vi "example.vi"() -> ()   [LabVIEW 2014]
uses:
  <vilib>/NI/TBM Modules/Sequencer/module/execution/Simple Sequencer TBM runtime.lvclass
  Code/3D Gears Demo/Source Code/actions/dwell/Dwell Config.lvclass
  <vilib>/NI/TBM Modules/Sequencer/module/configuration/Simple Sequencer TBM configuration.lvclass
  <vilib>/NI/TBM Modules/Sequencer/module/configuration/sequence definition.ctl
  <vilib>/NI/TBM Modules/Sequencer/sequencer parent classes/sequencer config parent/base TBM sequencer configuration.lvclass
  <vilib>/NI/Tag Bus Module Framework/channel/TBM channel.lvclass
  <vilib>/NI/Tag Bus/tag/Data Type.ctl
  <vilib>/NI/Tag Bus/tag/tag descriptor.lvclass
  <vilib>/NI/Tag Bus Module Framework/channel/channel classification.ctl
  <vilib>/NI/TBM Modules/Sequencer/sequencer parent classes/action configuration parent/action configuration.lvclass
  Code/3D Gears Demo/Source Code/actions/toggle/configuration/Toggle Config.lvclass
  Code/3D Gears Demo/Source Code/actions/dwell/runtime/Dwell.lvclass
  Code/3D Gears Demo/Source Code/actions/toggle/runtime/Toggle.lvclass
panel:
  out "error out":errorcluster
  in  "stop":bool
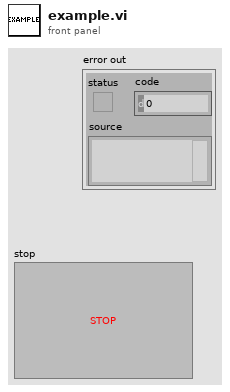
[diagram p1: front panel]
types:
  T1 = typedef "TBM channel.lvclass/channel classification.ctl" = enum16{"input data", "output data", "processing parameter", "processing result"}
  T2 = typedef "tag bus.lvlib/tag descriptor.lvclass/Data Type.ctl" = enum16{"Double", "Single", "I64", "I32", "I16", "I8", "U64", "U32", "U16", "U8", "Boolean", "String", "Array of Double", "Array of Single", "Array of I64", "Array of I32", "Array of I16", "Array of I8", "Array of U64", "Array of U32", "Array of U16", "Array of U8", "Array of Boolean", "Array of String"}
  T3 = typedef "Simple Sequencer TBM configuration.lvclass/sequence definition.ctl" = cluster{"sequence name":string, "action configs":refnum<class "action configuration.lvclass">[]}
  T4 = typedef "TBM channel.lvclass/data tables.ctl" = cluster{"input data":T5, "processing parameter":T5, "processing result":T5, "output data":T5}
  T5 = typedef "tag bus.lvlib/dictionary table pair.ctl" = cluster{"data dictionary":refnum<class "data dictionary.lvclass">, "data table":T6}
  T6 = typedef "tag bus.lvlib/data table.lvlib/data table.ctl" = cluster{"Double":dbl[], "Single":sgl[], "I64":i64[], "I32":i32[], "I16":i16[], "I8":i8[], "U64":u64[], "U32":u32[], "U16":u16[], "U8":u8[], "Boolean":bool[], "String":string[], "Array of Double":cluster{"DBL Array":dbl[]}[], "Array of Single":cluster{"SGL Array":sgl[]}[], "Array of I64":cluster{"I64 Array":i64[]}[], "Array of I32":cluster{"I32 Array":i32[]}[], "Array of I16":cluster{"I16 Array":i16[]}[], "Array of I8":cluster{"I8 Array":i8[]}[], "Array of U64":cluster{"U64 Array":u64[]}[], "Array of U32":cluster{"U32 Array":u32[]}[], "Array of U16":cluster{"U16 Array":u16[]}[], "Array of U8":cluster{"U8 Array":u8[]}[], "Array of Boolean":cluster{"Boolean Array":bool[]}[], "Array of String":cluster{"String Array":string[]}[]}
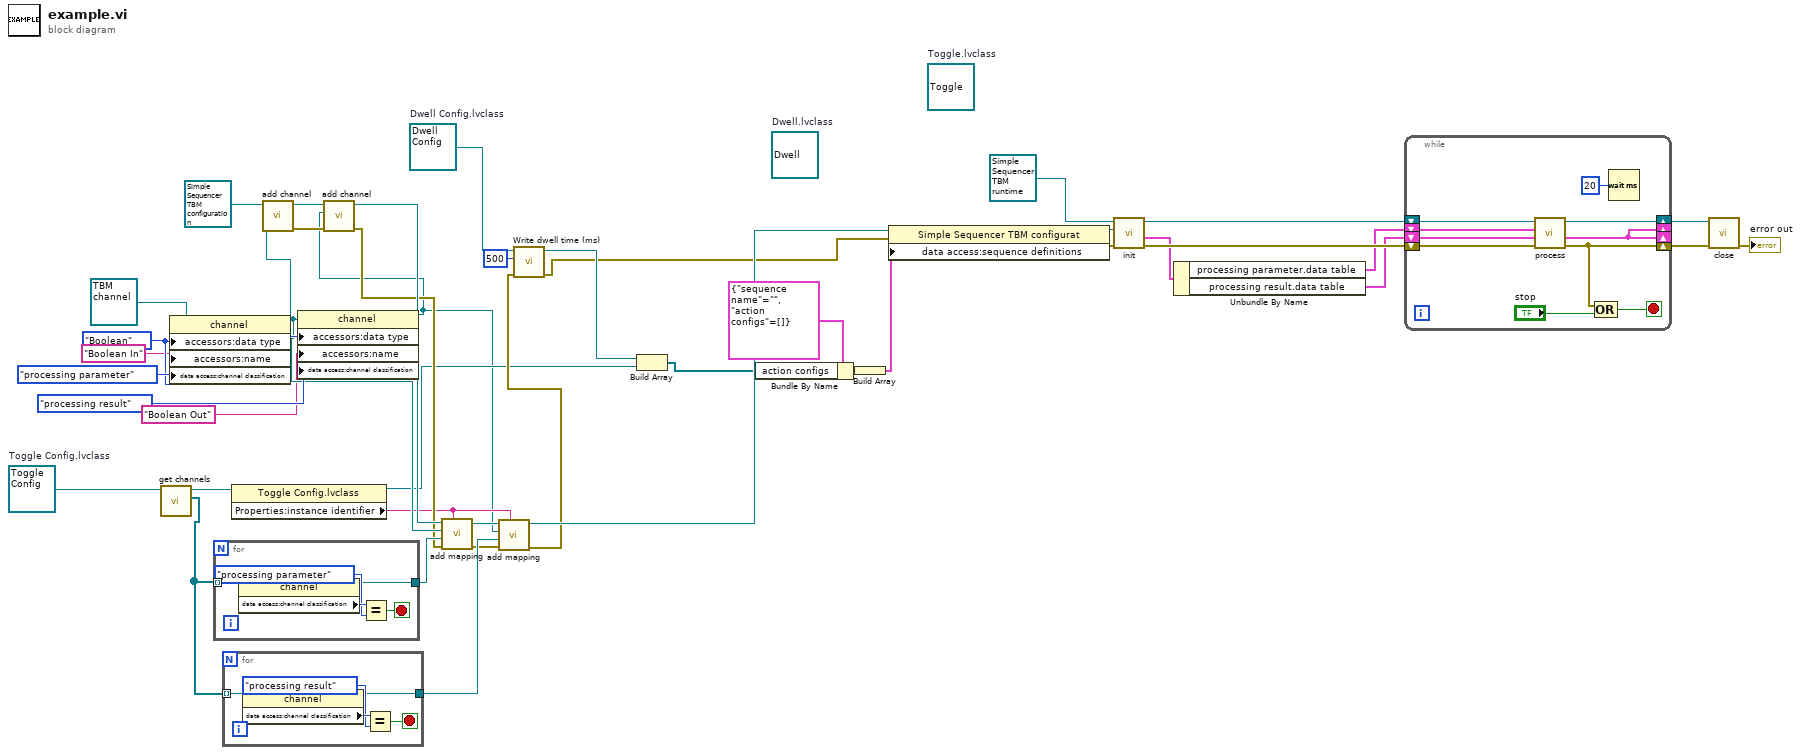
[diagram p0: block diagram]
diagram:
  (unwired) refnum<class "Toggle.lvclass"> refnum  # Toggle.lvclass
  (unwired) refnum<class "Dwell.lvclass"> refnum  # Dwell.lvclass
  w1 = refnum<class "Dwell Config.lvclass"> refnum  # Dwell Config.lvclass
  w2 = refnum<class "Toggle Config.lvclass"> refnum  # Toggle Config.lvclass
  w24 = Data_Type."Boolean" ("data type")
  n1 = call-dynamic "get channels.vi"("ActionCfg_Toggle in"=w2) -> ("action channels"=w13:refnum<class "TBM channel.lvclass">[], "ActionCfg_Toggle out"=w19:refnum<class "Toggle Config.lvclass">)  [unwired: 8 in, 1 out]
  n2 = property class="channel"(reference=refnum<class "TBM channel.lvclass"> refnum ("channel descriptor"), "accessors:data type"=w24, "accessors:name"="Boolean In" ("name"), "data access:channel classification"=channel_classification."processing parameter" ("channel classification")) -> (reference out=w18:refnum<class "TBM channel.lvclass">)  [unwired: 1 in, 1 out]
  n3 = for {
    tunnel: w13 -> [w48] mode=indexing
    tunnel: [w44] -> w17
    stop <- w45 stop-if-true
    n4 = property class="channel"(reference=w48) -> (reference out=w44:refnum<class "TBM channel.lvclass">, "data access:channel classification"=w47:T1)  [unwired: 1 in, 1 out]
    n5 = Equal?(x=w47, y=channel_classification."processing parameter") -> (x = y?=w45:bool)
  }
  n6 = for {
    tunnel: w13 -> [w53] mode=indexing
    tunnel: [w49] -> w12
    stop <- w50 stop-if-true
    n7 = property class="channel"(reference=w53) -> (reference out=w49:refnum<class "TBM channel.lvclass">, "data access:channel classification"=w52:T1)  [unwired: 1 in, 1 out]
    n8 = Equal?(x=w52, y=channel_classification."processing result") -> (x = y?=w50:bool)
  }
  n9 = property class="Toggle Config.lvclass"(reference=w19) -> (reference out=w7:refnum<class "Toggle Config.lvclass">, "Properties:instance identifier"=w8:string)  [unwired: 1 in, 1 out]
  n10 = call <vilib>:"add channel.vi"("channel descriptor"=w18, "engine configuration in"=refnum<class "Simple Sequencer TBM configuration.lvclass"> refnum ("Simple Sequencer TBM configuration")) -> ("error out"=w21:errorcluster, "engine configuration out"=w25:refnum<class "Simple Sequencer TBM configuration.lvclass">)  [unwired: 8 in]
  n11 = property class="channel"(reference=w18, "accessors:data type"=w24, "accessors:name"="Boolean Out" ("name"), "data access:channel classification"=channel_classification."processing result" ("channel classification")) -> (reference out=w6:refnum<class "TBM channel.lvclass">)  [unwired: 1 in, 1 out]
  n12 = call <vilib>:"add channel.vi"("error in"=w21, "channel descriptor"=w6, "engine configuration in"=w25) -> ("error out"=w10:errorcluster, "engine configuration out"=w20:refnum<class "Simple Sequencer TBM configuration.lvclass">)  [unwired: 7 in]
  n13 = call <vilib>:"add mapping.vi"("owner ID"=w8, "error in"=w10, "action channel"=w17, "seq channel"=w18, "engine configuration"=w20) -> ("error out"=w11:errorcluster, "engine configuration out"=w16:refnum<class "Simple Sequencer TBM configuration.lvclass">)  [unwired: 5 in]
  n14 = call <vilib>:"add mapping.vi"("owner ID"=w8, "error in"=w11, "action channel"=w12, "seq channel"=w6, "engine configuration"=w16) -> ("error out"=w9:errorcluster, "engine configuration out"=w15:refnum<class "Simple Sequencer TBM configuration.lvclass">)  [unwired: 5 in]
  n15 = call "Write dwell time (ms).vi"("error in (no error)"=w9, "dwell time (ms)"=u32 500, "ActionCfg_Dwell in"=w1) -> ("error out"=w4:errorcluster, "ActionCfg_Dwell out"=w5:refnum<class "Dwell Config.lvclass">)  [unwired: 7 in]
  n16 = Build Array(w5, w7) -> (w3:refnum<class "action configuration.lvclass">[])
  n17 = Bundle By Name(cluster=T3 {"sequence name"="", "action configs"=[]} ("sequence definitions"), "action configs"=w3) -> (w30:T3)
  n18 = Build Array(w30) -> (w29:T3[])
  n19 = property class="Simple Sequencer TBM configurat"(reference=w15, error in=w4, "data access:sequence definitions"=w29) -> (reference out=w34:refnum<class "Simple Sequencer TBM configuration.lvclass">, error out=w33:errorcluster)
  n20 = call-dynamic "init.vi"("error in"=w33, "module configuration"=w34, "Simple Sequencer TBM runtime in"=refnum<class "Simple Sequencer TBM runtime.lvclass"> refnum) -> ("error out"=w43:errorcluster, "data allocations"=w40:T4, "Simple Sequencer TBM runtime out"=w41:refnum<class "Simple Sequencer TBM runtime.lvclass">)  [unwired: 5 in, 1 out]
  n21 = Unbundle By Name(w40) -> ("processing parameter.data table"=w39:T6, "processing result.data table"=w38:T6)
  n22 = while {
    shift-right: [w57] -> w42
    shift-left: w43 -> [w62]
    shift-right: [w61] -> w36
    shift-left: w41 -> [w60]
    shift-right: [w54] -> _
    shift-left: w39 -> [w55]
    shift-right: [w54] -> _
    shift-left: w38 -> [w59]
    stop <- w56 stop-if-true
    n23 = call-dynamic "process.vi"("error in"=w62, "result allocation"=w59, "parameters"=w55, "Simple Sequencer TBM runtime in"=w60) -> ("error out"=w57:errorcluster, "results"=w54:T6, "Simple Sequencer TBM runtime out"=w61:refnum<class "Simple Sequencer TBM runtime.lvclass">)  [unwired: 4 in, 1 out]
    n24 = Compound Arithmetic op=OR(w57, "stop") -> (w56:bool)
    n25 = Wait (ms)(milliseconds to wait=u32 20) -> ()  [unwired: 1 out]
  }
  n26 = call-dynamic "close.vi"("error in"=w42, "Simple Sequencer TBM runtime in"=w36) -> ("error out"=→"error out":errorcluster)  [unwired: 9 in]
